vi "Washer Read.vi"(0 "Com Chan":u8, 1 "Partial Message Start":u8[](array[numeric]) format="%02x", 7 "Washer Data In":T1, 11 "error in (no error)":errorcluster) -> (4 "Washer Data Out":T1, 6 "Read Buffer":string, 8 "Log String":string, 10 "Partial Message Out":u8[](array[numeric]) format="%.0x", 15 "error out":errorcluster)   [LabVIEW 2011]
uses:
  HCC Data.ctl
  Washer Status Ctrl.ctl
  GEA2 Washer Interface Ctrl.ctl
  Globals HCC.vi
panel:
  out "Debug Log":string
  out "Good Responses":cluster{"Bytes Data":u8[]}[](array[cluster])
  out "x-y":u32
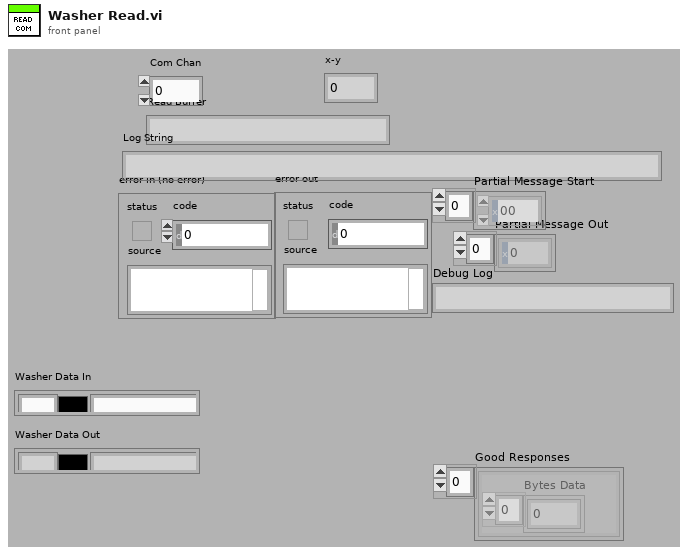
[diagram p1: front panel]
types:
  T1 = typedef "HCC Data.ctl" = cluster{"Station":string, "Color":u32, "Status":T2, "Error Time":string, "Com Err Count":u32, "Debug Log":string}
  T2 = typedef "Washer Status Ctrl.ctl" = enum16{"Running", "Err", "No Com", "No Conf"}
  T3 = typedef "GEA2 Washer Interface Ctrl.ctl" = enum16{"Init Com Port", "SendCMD", "ReadPort", "Close Port", "Send Byte Data", "Read Continuous"}
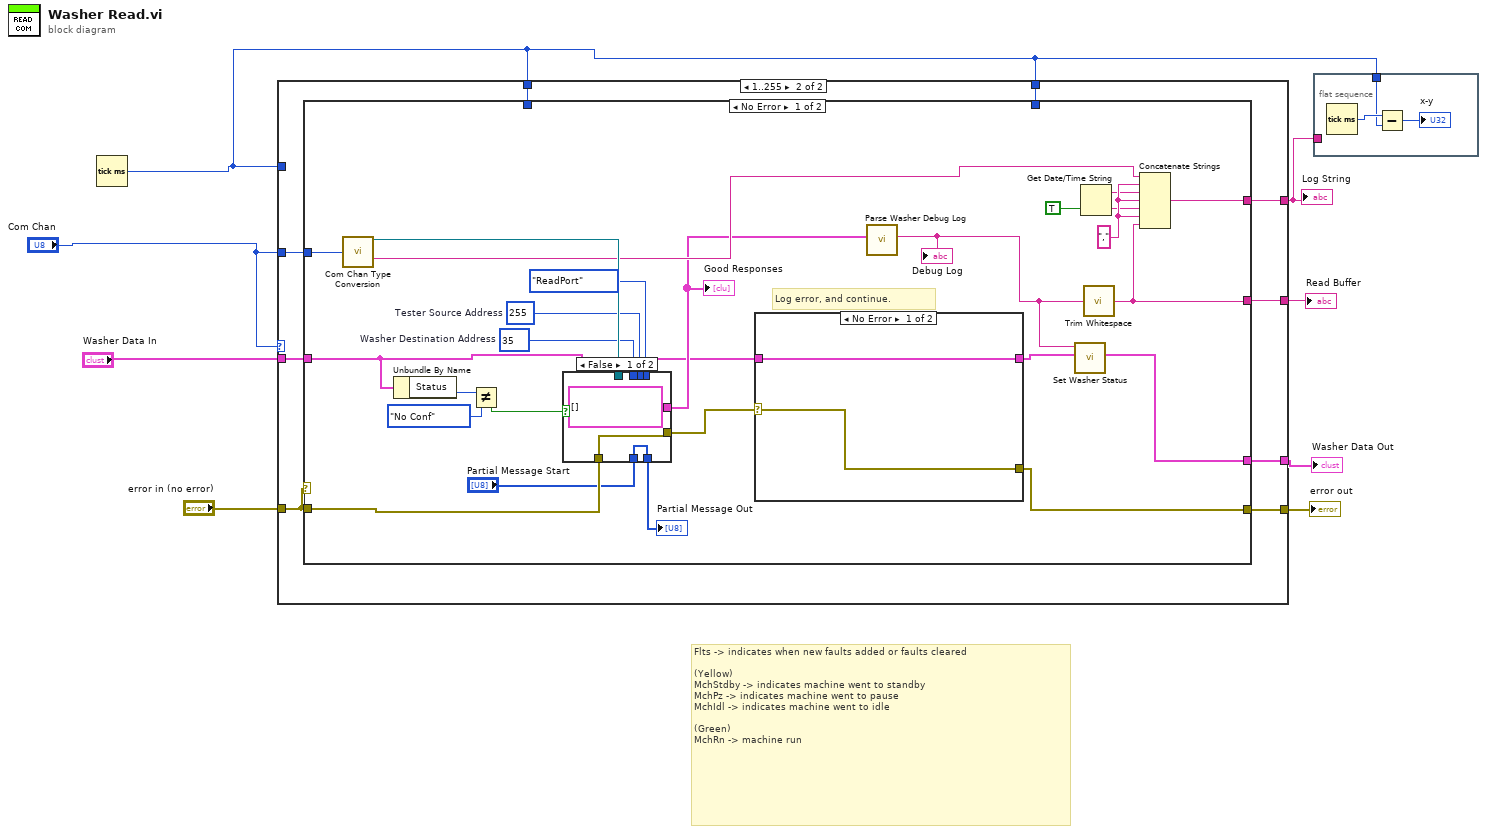
[diagram p0: block diagram]
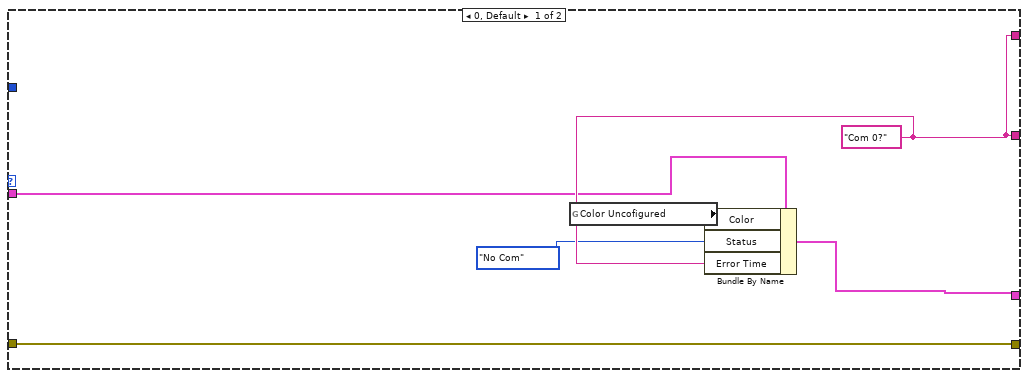
[diagram p2: hidden frame]
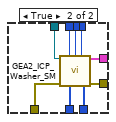
[diagram p3: hidden frame]
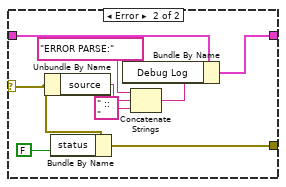
[diagram p4: hidden frame]
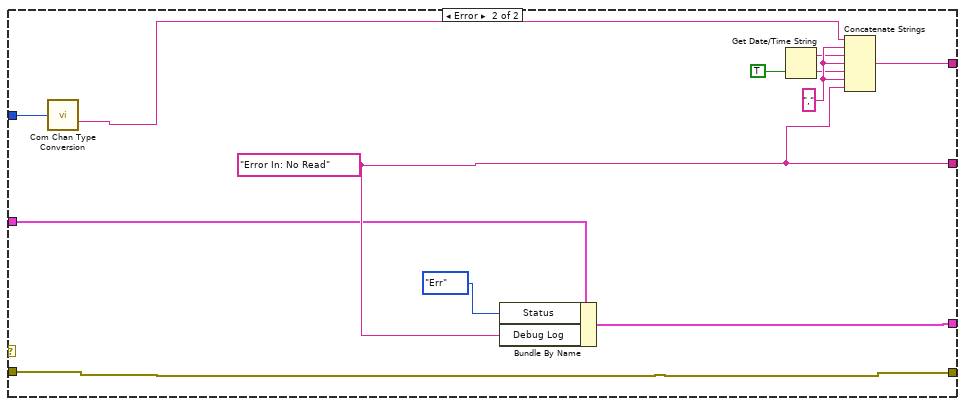
[diagram p5: hidden frame]
diagram:
  # "Flts -> indicates when new faults added or faults cleared\n\n(Yellow)\nMchStdby -> indicates machine went to standby\nMchPz -> indicates machine went to pause\nMchIdl -> indicates machine went to idle \n\n(Green)\nMchRn -> machine run"
  n1 = Tick Count (ms)() -> (millisecond timer value=w3:u32)
  n2 = case shown="1..255" "Com Chan" {
    tunnel: "Com Chan" -> [_ w23]
    tunnel: [w14 w22] -> w8
    tunnel: "error in (no error)" -> [w14 w21]
    tunnel: [w12 w20] -> w4
    tunnel: [w12 w19] -> w5
    tunnel: [w11 w18] -> w1
    tunnel: "Washer Data In" -> [w10 w17]
    tunnel: w3 -> [_ _]
    tunnel: w3 -> [_ w16]
    tunnel: w3 -> [_ w15]
    frame 0, Default {
      w12 = "Com 0?" ("ASCII Data")
      n3 = global read "Globals HCC.vi" "Color Uncofigured"() -> (w13:u32)
      n4 = Bundle By Name(cluster=w10, "Color"=w13, "Status"=Washer_Status_Ctrl."No Com", "Error Time"=w12) -> (w11:T1)
    }
    frame 1..255 {
      n5 = case shown="No Error" w21 {
        tunnel: w23 -> [w41 w77]
        tunnel: [w48 w83] -> w22
        tunnel: w21 -> [w47 w83]
        tunnel: [w40 w76] -> w20
        tunnel: [w39 w75] -> w19
        tunnel: [w31 w74] -> w18
        tunnel: w17 -> [w27 w73]
        tunnel: w16 -> [_ _]
        tunnel: w15 -> [_ _]
        frame No Error {
          w29 = u8 255  # Tester Source Address
          w28 = u8 35  # Washer Destination Address
          w45 = "," ("string")
          # "Log error, and continue."
          n6 = call "Com Chan Type Conversion.vi"("Com Chan"=w41) -> ("VISA resource name"=w46:refnum<visa-resource-name>, "Com Text"=w34:string)  [unwired: 11 in, 2 out]
          n7 = Unbundle By Name(w27) -> ("Status"=w26:T2)
          n8 = Not Equal?(x=w26, y=Washer_Status_Ctrl."No Conf" ("Status")) -> (x != y?=w24:bool)
          n9 = case shown="False" w24 {
            tunnel: w47 -> [w50 w60]
            tunnel: w46 -> [_ w59]
            tunnel: [w50 w58] -> w38
            tunnel: "Partial Message Start" -> [w49 w57]
            tunnel: [w49 w56] -> w36
            tunnel: GEA2_Washer_Interface_Ctrl."ReadPort" ("Mode") -> [_ w55]
            tunnel: [cluster{"Bytes Data":u8[]}[] [] ("Good Responses") w54] -> w33
            tunnel: w29 -> [_ w53]
            tunnel: w28 -> [_ w52]
            frame False {
            }
            frame True {
              n10 = call "GEA2_ICP_Washer_SM.vi"("ComPort"=w59, "Destination Address"=w52, "Source Address"=w53, "Mode"=w55, "Error In"=w60, "Partial Message Start"=w57) -> ("Good Responses"=w54:cluster{"Bytes Data":u8[]}[], "Partial Message Out"=w56:u8[], "Error Out"=w58:errorcluster)  [unwired: 6 in, 1 out]
            }
          }
          "Partial Message Out" <- w36
          "Good Responses" <- w33
          n11 = case shown="No Error" w38 {
            selector: w38 -> [w62 w66]
            tunnel: [w61 w63] -> w32
            tunnel: [w62 w67] -> w48
            tunnel: w27 -> [w61 w64]
            frame No Error {
            }
            frame Error {
              n12 = Unbundle By Name(w66) -> ("source"=w69:string)
              n13 = Bundle By Name(cluster=w66, "status"=FALSE) -> (w67:errorcluster)
              n14 = Concatenate Strings("ERROR PARSE:" ("string"), w69, " :: " ("string")) -> (w71:string)
              n15 = Bundle By Name(cluster=w64, "Debug Log"=w71) -> (w63:T1)
            }
          }
          n16 = call "Parse Washer Debug Log.vi"("Good Responses"=w33) -> ("Debug Log"=w30:string)  [unwired: 10 in]
          "Debug Log" <- w30
          n17 = call "Set Washer Status.vi"("Washer Data In"=w32, "Debug Log"=w30) -> ("Washer Data Out"=w31:T1)  [unwired: 9 in]
          n18 = Get Date/Time String(want seconds? (F)=TRUE) -> (date string=w43:string, time string=w44:string)  [unwired: 2 in]
          n19 = call <vilib>:"Trim Whitespace.vi"("string"=w30) -> ("trimmed string"=w39:string)  [unwired: 1 in]
          n20 = Concatenate Strings(w34, w45, w43, w45, w44, w45, w39) -> (w40:string)
        }
        frame Error {
          w75 = "Error In: No Read" ("ASCII Data")
          w82 = "," ("string")
          n21 = call "Com Chan Type Conversion.vi"("Com Chan"=w77) -> ("Com Text"=w78:string)  [unwired: 11 in, 3 out]
          n22 = Bundle By Name(cluster=w73, "Status"=Washer_Status_Ctrl."Err", "Debug Log"=w75) -> (w74:T1)
          n23 = Get Date/Time String(want seconds? (F)=TRUE) -> (date string=w80:string, time string=w81:string)  [unwired: 2 in]
          n24 = Concatenate Strings(w78, w82, w80, w82, w81, w82, w75) -> (w76:string)
        }
      }
    }
  }
  "error out" <- w8
  "Log String" <- w4
  "Read Buffer" <- w5
  "Washer Data Out" <- w1
  n25 = flat-sequence {
    tunnel: w4 -> [_]
    tunnel: w3 -> [w85]
    frame #0 {
      n26 = Tick Count (ms)() -> (millisecond timer value=w86:u32)
      n27 = Subtract(x=w86, y=w85) -> (x-y=→"x-y":u32)
    }
  }
